vi "FPGA Main V2.vi"() -> ()   [LabVIEW 2018]
doc: "This VI reads all analogue data channels available at the fastest rate supported by the respective hardware and updates a memory address for when each measurement is available.\n\nAt a rate defined by the fastest module (NI 9237 - default of 12.5kHz) this memory is read, combined with the measurements from the 9237 module and written to the FIFO for communication to the RT machine.\n\nThe NI 9237 modeul therefore defines the nominal sampling rate of the system (with slower channels over-sampled).\n\nA time channel (in uSec) is provided with 0 referenced from the first acquisition of the NI 9237 module"
uses:
  <vilib>/LabVIEW Targets/FPGA/cRIO/shared/nicrio_ModuleControls/nicrio_cRIO-9237_DataRatesRing.ctl
  <vilib>/Platform/TimedLoop/XDataNode/timing_clust.ctl
  <vilib>/Platform/TimedLoop/XDataNode/nitl_modes.ctl
  <vilib>/Platform/TimedLoop/XDataNode/wakeup.ctl
  <vilib>/rvi/Emulation/niFpgaGetClockAttributes.vi
  <vilib>/rvi/Emulation/niFpgaSctlEmulationGetInTimedLoop.vi
  <vilib>/rvi/Emulation/niFpgaEmulationReportErrorSimple.vi
  <vilib>/rvi/Emulation/niFpgaProcessEmulError.vi
  <vilib>/rvi/eio/common/nirviEmuTemplatePropertySet_noerrors.vi
  <vilib>/rvi/eio/common/nirviEmuTemplateMethod_errors.vi
  <vilib>/rvi/interface/RandomDataEmulation/niFpgaRandomDataHandleErrors.vi
  <vilib>/rvi/Memory/Memory_Emulation/nirvimemoryFastEmulation.vi
  <vilib>/rvi/Memory/Memory_Emulation/nirvimemoryEmulation.vi
  <vilib>/rvi/Emulation/niFpgaEmulationIsFPGAContextNoSignature.vi
  <vilib>/rvi/DataTransferAndStorage/Container/Common/niFpgaContainerGetUniqueNameForEmu.vi
  <vilib>/rvi/errors/nirviReportUnexpectedCaseInternalError (U32).vi
  <vilib>/rvi/Emulation/niFpgaCriticalErrorInLSC.vi
  <vilib>/eio/EIOPropertyNode/EIOPropertyNode.xnode
  <vilib>/eio/EIONode/EIONode.xnode
  <vilib>/rvi/DataTransferAndStorage/Container/XNode/niFpgaContainer.xnode
  <vilib>/rvi/interface/RandomDataEmulation/nirviRandomDataFpgaReadWriteTemplate.vi
  <vilib>/platform/TimedLoop/XDataNode/XDataNode.xnode
  <vilib>/eio/EIOMethodNode/EIOMethodNode.xnode
  <vilib>/Platform/TimedLoop/XDataNode/XDNodeRunTimeDep.lvlib
  <vilib>/rvi/eio/common/nirviEmuTemplatePropertyGet_errors.vi
  <vilib>/rvi/eio/common/nirviEmuTemplatePropertyGet_noerrors.vi
  <vilib>/rvi/eio/common/nirviEmuTemplatePropertySet_errors.vi
panel:
  in  "speedDirection":bool=TRUE
  in  "speed filter":u16=150
  in  "switch encoders":bool
  in  "falling edge (F)":bool caption="Torque encoder direction"
  in  "filterTorque":bool
  in  "Data Rate":T1=1 items=["50.000 kS/s (NI 9237)"=1, "25.000 kS/s (NI 9237)"=2, "16.667 kS/s (NI 9237)"=3, "12.500 kS/s (NI 9237)"=4, "10.000 kS/s (NI 9237)"=5, "8.333 kS/s (NI 9237)"=6, "7.143 kS/s (NI 9237)"=7, "6.250 kS/s (NI 9237)"=8, "5.556 kS/s (NI 9237)"=9, "5.000 kS/s (NI 9237)"=10, "4.545 kS/s (NI 9237)"=11, "4.167 kS/s (NI 9237)"=12, "3.846 kS/s (NI 9237)"=13, "3.571 kS/s (NI 9237)"=14, "3.333 kS/s (NI 9237)"=15, "3.125 kS/s (NI 9237)"=16, "2.941 kS/s (NI 9237)"=17, "2.778 kS/s (NI 9237)"=18, "2.632 kS/s (NI 9237)"=19, "2.500 kS/s (NI 9237)"=20, "2.381 kS/s (NI 9237)"=21, "2.273 kS/s (NI 9237)"=22, "2.174 kS/s (NI 9237)"=23, "2.083 kS/s (NI 9237)"=24, "2.000 kS/s (NI 9237)"=25, "1.923 kS/s (NI 9237)"=26, "1.852 kS/s (NI 9237)"=27, "1.786 kS/s (NI 9237)"=28, "1.724 kS/s (NI 9237)"=29, "1.667 kS/s (NI 9237)"=30, "1.613 kS/s (NI 9237)"=31]
  in  "encoders offset":sgl caption="encoder offset (radians)"
  out "Total channel count":u32=61
  out "timestamp":u32
  out "FIFO full counter":i32
  in  "Safe Voltage":fxp<+/-,20,5>[](array[numeric])=[0.0, 0.0, 0.0, 0.0]
  in  "Safe Digital":bool[](array[boolean])=[FALSE, FALSE, FALSE, FALSE, FALSE, FALSE, FALSE, FALSE]
  in  "Voltage Out":fxp<+/-,20,5>[](array[numeric])=[0.0, 0.0, 0.0, 0.0]
  in  "Update Outputs":bool
  in  "Mod 8":bool[](array[boolean])=[FALSE, FALSE, FALSE, FALSE, FALSE, FALSE, FALSE, FALSE]
  out "E Stop":bool
  in  "Stop acquire":bool
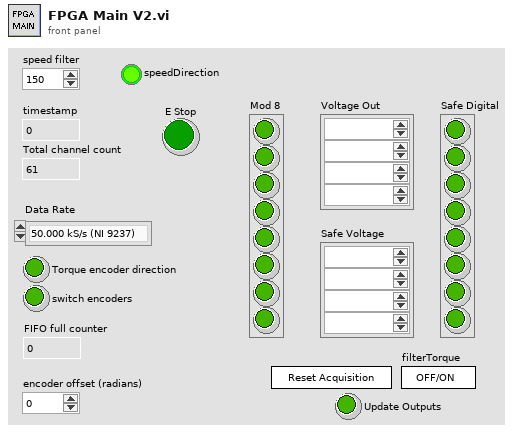
[diagram p1: front panel]
types:
  T1 = typedef "nicrio_cRIO-9237_DataRatesRing.ctl" = u8
  T2 = typedef "XDNodeRunTimeDep.lvlib/timing_clust.ctl" = cluster{"Expected End [f-1]":u64, "Actual End [f-1]":u64, "Finished Late? [f-1]":bool, "Expected End [i-1]":u64, "Actual End [i-1]":u64, "Finished Late? [i-1]":bool, "Expected Start [i]":u64, "Actual Start [i]":u64, "Expected Start [f]":u64, "Actual Start [f]":u64, "Source Name":string, "Structure Name":string, "Period":i64, "Deadline":i64, "Offset":i64, "Start":i64, "Priority":i32, "Timeout":i32, "Mode":T3, "Wakeup Reason":T4, "Error":errorcluster, "Source Type":string, "Secondary Source Type":string, "Global End Time":u64, "Global Start Time":u64, "Frame Duration":u64, "Iteration Duration":u64, "Assigned CPU":i32, "I/O Scan Engine Mode":u32}
  T3 = typedef "XDNodeRunTimeDep.lvlib/nitl_modes.ctl" = enum32{"No Change", "Process missed periods, maintain original phase", "Discard missed periods, maintain original phase", "Process missed periods, ignore original phase", "Discard missed periods, ignore original phase"}
  T4 = typedef "XDNodeRunTimeDep.lvlib/wakeup.ctl" = enum32{"Normal", "Aborted", "Asynchronous wakeup", "Timing source error", "Timed loop error", "Timeout"}
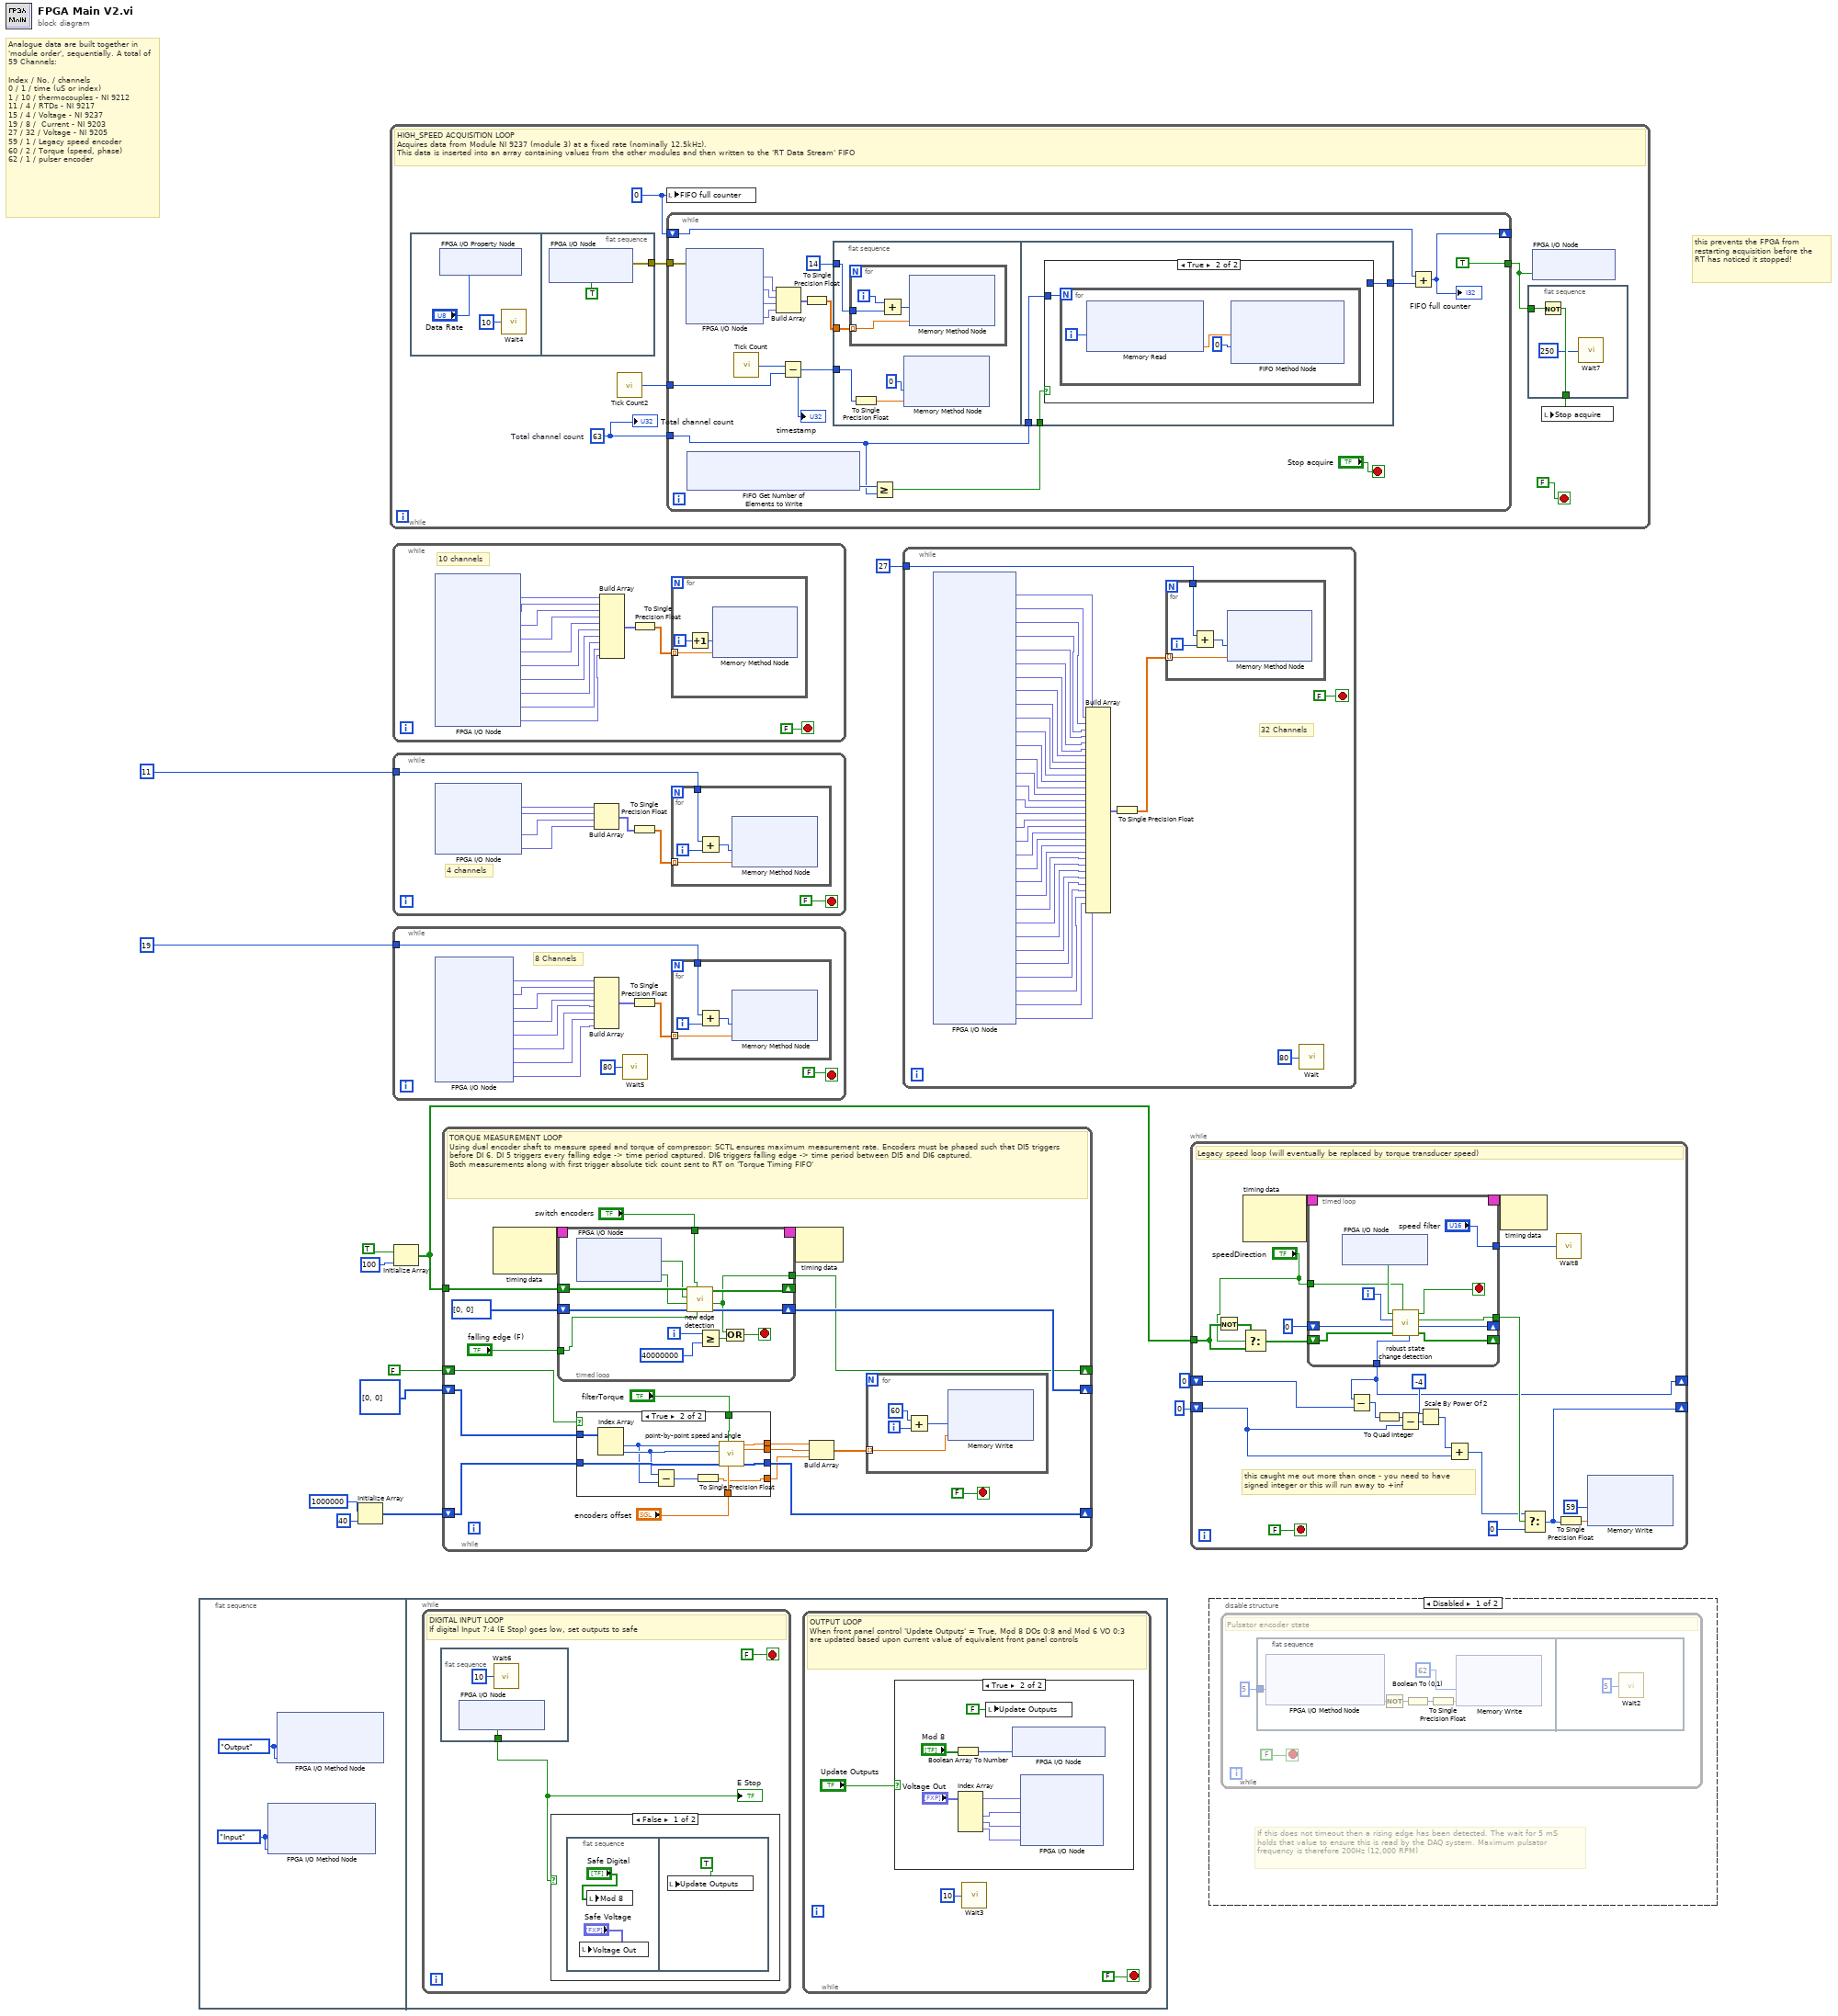
[diagram p0: block diagram]
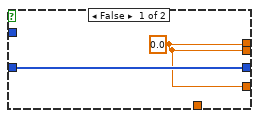
[diagram p5: hidden frame]
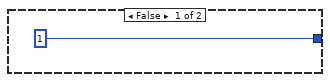
[diagram p6: hidden frame]
diagram:
  # "this prevents the FPGA from restarting acquisition before the RT has noticed it stopped!"
  # "Analogue data are built together in 'module order', sequentially. A total of 59 Channels:\n\nIndex / No. / channels\n0 / 1 / time (uS or index)\n1 / 10 / thermocouples - NI 9212\n11 / 4 / RTDs - NI 9217\n15 / 4 / Voltage - NI 9237\n19 / 8 /  Current - NI 9203\n27 / 32 / Voltage - NI 9205\n59 / 1 / Legacy speed encoder\n60 / 2 / Torque (speed, phase)\n62 / 1 / pulser encoder"
  n1 = flat-sequence {
    frame #0 {
      w14 = enum8{"No Change", "Input", "Output"}."Output" ("DIO 7:4")
      w15 = enum8{"No Change", "Input", "Output"}."Input" ("DIO 7:4")
      n2 = xnode "FPGA I/O Method Node"("DIO 7:4"=w15, "DIO 3:0"=w15) -> ()  [unwired: 1 in, 1 out]
      n3 = xnode "FPGA I/O Method Node"("DIO 7:4"=w14, "DIO 3:0"=w14) -> ()  [unwired: 1 in, 1 out]
    }
    frame #1 {
      n4 = while {
        stop <- FALSE stop-if-true
        # "DIGITAL INPUT LOOP\nIf digital Input 7:4 (E Stop) goes low, set outputs to safe"
        n5 = flat-sequence {
          tunnel: [w30] -> w27
          frame #0 {
            n6 = xnode "FPGA I/O Node"() -> ("Mod7/DIO4"=w30:bool)  [unwired: 1 in, 1 out]
            n7 = call "Wait6"("Count(uSec)"=u8 10) -> ()  [unwired: 1 out]
          }
        }
        n8 = case shown="False" w27 {
          frame False {
            n9 = flat-sequence {
              frame #0 {
                n10 = local write "Voltage Out"("Safe Voltage") -> ()
                n11 = local write "Mod 8"("Safe Digital") -> ()
              }
              frame #1 {
                n12 = local write "Update Outputs"(TRUE ("Update Outputs")) -> ()
              }
            }
          }
          frame True {
          }
        }
        "E Stop" <- w27
      }
      n13 = while {
        stop <- FALSE stop-if-true
        # "OUTPUT LOOP\nWhen front panel control 'Update Outputs' = True, Mod 8 DOs 0:8 and Mod 6 VO 0:3 are updated based upon current value of equivalent front panel controls"
        n14 = case shown="True" "Update Outputs" {
          frame False {
          }
          frame True {
            n15 = Boolean Array To Number(Boolean array="Mod 8") -> (number=w25:u8)
            n16 = Index Array(array="Voltage Out") -> (element #1=w23:fxp<+/-,20,5>, element #2=w22:fxp<+/-,20,5>, element #3=w21:fxp<+/-,20,5>, element #4=w20:fxp<+/-,20,5>)  [unwired: 4 in]
            n17 = local write "Update Outputs"(FALSE ("Update Outputs")) -> ()
            n18 = xnode "FPGA I/O Node"("Mod8/DIO7:0"=w25) -> ()  [unwired: 1 in, 1 out]
            n19 = xnode "FPGA I/O Node"("Mod6/AO0"=w23, "Mod6/AO1"=w22, "Mod6/AO2"=w21, "Mod6/AO3"=w20) -> ()  [unwired: 4 in, 4 out]
          }
        }
        n20 = call "Wait3"("Count(uSec)"=u16 10 ("Count(Ticks)")) -> ()  [unwired: 1 out]
      }
    }
  }
  n21 = Initialize Array(u32 1000000 ("64bit integer"), 40 ("dimension size")) -> (w8:u32[])
  n22 = while {
    stop <- FALSE stop-if-true
    w35 = 0 ("FIFO full counter")
    w38 = u32 63  # Total channel count
    # "HIGH_SPEED ACQUISITION LOOP\nAcquires data from Module NI 9237 (module 3) at a fixed rate (nominally 12.5kHz).\nThis data is inserted into an array containing values from the other modules and then written to the 'RT Data Stream' FIFO"
    n23 = flat-sequence {
      tunnel: [w47] -> w39
      frame #0 {
        n24 = xnode "FPGA I/O Property Node"("Data Rate"="Data Rate") -> ()  [unwired: 1 in, 1 out]
        n25 = call "Wait4"("Count(mSec)"=u16 10) -> ()  [unwired: 1 out]
      }
      frame #1 {
        n26 = xnode "FPGA I/O Node"("Mod3/Start"=TRUE) -> ("error out"=w47:errorcluster)  [unwired: 2 in, 1 out]
      }
    }
    n27 = call "Tick Count2"() -> ("Tick Count(uSec)"=w40:u32)
    n28 = local write "FIFO full counter"(w35) -> ()
    n29 = while {
      tunnel: [TRUE ("I/O Item")] -> w37
      tunnel: w39 -> [w65]
      tunnel: w38 -> [w50]
      shift-right: [w58] -> _
      shift-left: w35 -> [w56]
      tunnel: w40 -> [w59]
      stop <- "Stop acquire" stop-if-true
      n30 = xnode "FPGA I/O Node"("error in"=w65) -> ("Mod3/AI0"=w64:fxp<+/-,24,-4>, "Mod3/AI1"=w63:fxp<+/-,24,-4>, "Mod3/AI2"=w62:fxp<+/-,24,-4>, "Mod3/AI3"=w61:fxp<+/-,24,-4>)  [unwired: 4 in, 5 out]
      n31 = xnode ("FIFO Get Number of Elements to Write")() -> ("Number of Elements to Write"=w52:u32)  [unwired: 1 in, 1 out]
      n32 = call "Tick Count"() -> ("Tick Count(uSec)"=w55:u32)
      n33 = Build Array(w64, w63, w62, w61) -> (w60:fxp<+/-,24,-4>[])
      n34 = Subtract(x=w55, y=w59) -> (x-y=w48:u32)
      "timestamp" <- w48
      n35 = To Single Precision Float(number=w60) -> (single precision float=w54:sgl[])
      n36 = flat-sequence {
        tunnel: w54 -> [w71]
        tunnel: 14 ("index") -> [w70]
        tunnel: w48 -> [w68]
        tunnel: w50 -> [w78]
        tunnel: [w77] -> w49
        tunnel: w51 -> [w76]
        frame #0 {
          n37 = for {
            tunnel: w71 -> [w75] mode=indexing
            tunnel: w70 -> [w74]
            i -> [w72]
            n38 = Add(x=w72, y=w74) -> (x+y=w73:i32)
            n39 = xnode ("Memory Method Node")("Address"=w73, "Data"=w75) -> ()  [unwired: 1 in, 1 out]
          }
          n40 = To Single Precision Float(number=w68) -> (single precision float=w69:sgl)
          n41 = xnode ("Memory Method Node")("Address"=u32 0, "Data"=w69) -> ()  [unwired: 1 in, 1 out]
        }
        frame #1 {
          n42 = case shown="True" w76 {
            tunnel: [1 _] -> w77
            tunnel: w78 -> [_ w80]
            frame False {
            }
            frame True {
              n43 = for {
                N: w80 -> [_]
                i -> [w81]
                n44 = xnode ("Memory Read")("Address"=w81) -> ("Data"=w82:sgl)  [unwired: 1 in, 1 out]
                n45 = xnode ("FIFO Method Node")("Element"=w82, "Timeout"=0) -> ()  [unwired: 1 in, 2 out]
              }
            }
          }
        }
      }
      n46 = Greater Or Equal?(x=w52, y=w50) -> (x >= y?=w51:bool)
      n47 = Add(x=w56, y=w49) -> (x+y=w58:i32)
      "FIFO full counter" <- w58
    }
    n48 = flat-sequence {
      tunnel: w37 -> [w43]
      tunnel: [w42] -> w34
      frame #0 {
        n49 = Not(x=w43) -> (.not. x?=w42:bool)
        n50 = call "Wait7"("Count(mSec)"=u8 250) -> ()  [unwired: 1 out]
      }
    }
    n51 = xnode "FPGA I/O Node"("Mod3/Stop"=w37) -> ()  [unwired: 1 in, 1 out]
    n52 = local write "Stop acquire"(w34) -> ()
    "Total channel count" <- w38
  }
  n53 = while {
    stop <- FALSE stop-if-true
    # "10 channels"
    n54 = xnode "FPGA I/O Node"() -> ("Mod1/TC0"=w96:fxp<+/-,24,-2>, "Mod1/TC1"=w95:fxp<+/-,24,-2>, "Mod1/TC2"=w94:fxp<+/-,24,-2>, "Mod1/TC3"=w93:fxp<+/-,24,-2>, "Mod1/TC4"=w92:fxp<+/-,24,-2>, "Mod1/TC5"=w91:fxp<+/-,24,-2>, "Mod1/TC6"=w90:fxp<+/-,24,-2>, "Mod1/TC7"=w89:fxp<+/-,24,-2>, "Mod1/CJC0"=w86:fxp<+/-,24,-2>, "Mod1/CJC1"=w85:fxp<+/-,24,-2>)  [unwired: 10 in, 10 out]
    n55 = Build Array(w96, w95, w94, w93, w92, w91, w90, w89, w86, w85) -> (w88:fxp<+/-,24,-2>[])
    n56 = To Single Precision Float(number=w88) -> (single precision float=w87:sgl[])
    n57 = for {
      tunnel: w87 -> [w99] mode=indexing
      i -> [w98]
      n58 = Increment(x=w98) -> (x+1=w97:i32)
      n59 = xnode ("Memory Method Node")("Address"=w97, "Data"=w99) -> ()  [unwired: 1 in, 1 out]
    }
  }
  n60 = while {
    tunnel: 11 ("Numeric") -> [w101]
    stop <- FALSE stop-if-true
    # "4 channels"
    n61 = xnode "FPGA I/O Node"() -> ("Mod2/RTD0"=w107:fxp<+/-,24,10>, "Mod2/RTD1"=w106:fxp<+/-,24,10>, "Mod2/RTD2"=w105:fxp<+/-,24,10>, "Mod2/RTD3"=w102:fxp<+/-,24,10>)  [unwired: 4 in, 4 out]
    n62 = Build Array(w107, w106, w105, w102) -> (w104:fxp<+/-,24,10>[])
    n63 = To Single Precision Float(number=w104) -> (single precision float=w103:sgl[])
    n64 = for {
      tunnel: w103 -> [w111] mode=indexing
      tunnel: w101 -> [w108]
      i -> [w110]
      n65 = Add(x=w108, y=w110) -> (x+y=w109:i32)
      n66 = xnode ("Memory Method Node")("Address"=w109, "Data"=w111) -> ()  [unwired: 1 in, 1 out]
    }
  }
  n67 = while {
    tunnel: 19 ("Numeric") -> [w118]
    stop <- FALSE stop-if-true
    # "8 Channels"
    n68 = xnode "FPGA I/O Node"() -> ("Mod4/AI0"=w124:fxp<+/-,21,-4>, "Mod4/AI1"=w123:fxp<+/-,21,-4>, "Mod4/AI2"=w122:fxp<+/-,21,-4>, "Mod4/AI3"=w119:fxp<+/-,21,-4>, "Mod4/AI4"=w117:fxp<+/-,21,-4>, "Mod4/AI5"=w116:fxp<+/-,21,-4>, "Mod4/AI6"=w115:fxp<+/-,21,-4>, "Mod4/AI7"=w114:fxp<+/-,21,-4>)  [unwired: 8 in, 8 out]
    n69 = Build Array(w124, w123, w122, w119, w117, w116, w115, w114) -> (w121:fxp<+/-,21,-4>[])
    n70 = call "Wait5"("Count(uSec)"=u8 80) -> ()  [unwired: 1 out]
    n71 = To Single Precision Float(number=w121) -> (single precision float=w120:sgl[])
    n72 = for {
      tunnel: w120 -> [w128] mode=indexing
      tunnel: w118 -> [w125]
      i -> [w127]
      n73 = Add(x=w125, y=w127) -> (x+y=w126:i32)
      n74 = xnode ("Memory Method Node")("Address"=w126, "Data"=w128) -> ()  [unwired: 1 in, 1 out]
    }
  }
  n75 = Initialize Array(TRUE, 100 ("edge buffer size")) -> (w4:bool[])
  n76 = while {
    shift-right: [w145] -> _
    shift-left: w8 -> [w146]
    tunnel: w4 -> [w144]
    shift-right: [w132] -> _
    shift-left: u32[] [0, 0] ("step") -> [w131]
    shift-right: [w129] -> _
    shift-left: FALSE ("edge detected") -> [w130]
    stop <- FALSE stop-if-true
    # "TORQUE MEASUREMENT LOOP\nUsing dual encoder shaft to measure speed and torque of compressor: SCTL ensures maximum measurement rate. Encoders must be phased such that DI5 triggers before DI 6. DI 5 triggers every falling edge -> time period captured. DI6 triggers falling edge -> time period between DI5 and DI6 captured.\nBoth measurements along with first trigger absolute tick count sent to RT on 'Torque Timing FIFO'"
    n77 = node-c288() -> (w142:T2)  [unwired: 2 in]
    n78 = timed-loop {
      timing: w142 -> [_]
      timing-out: [_] -> w141
      shift-right: [w171] -> _
      shift-left: w144 -> [w174]
      shift-right: [w172] -> w132
      shift-left: u32[] [0, 0] ("step") -> [w173]
      tunnel: "falling edge (F)" -> [w168]
      tunnel: [w169] -> w129
      tunnel: "switch encoders" -> [w165]
      i -> [w177]
      stop <- w170 stop-if-true
      n79 = xnode "FPGA I/O Node"() -> ("Mod7/DIO0"=w167:bool, "Mod7/DIO1"=w166:bool)  [unwired: 2 in, 2 out]
      n80 = call "new edge detection.vi"("rising edge (T)"=w168, "switch encoders (F)"=w165, "ticks"=w173, "encoder 2"=w166, "encoder 1"=w167, "history in"=w174) -> ("ticks out"=w172:u32[], "edge detected"=w169:bool, "history out"=w171:bool[])  [unwired: 3 in]
      n81 = Greater Or Equal?(x=w177, y=40000000) -> (x >= y?=w175:bool)
      n82 = Or(x=w169, y=w175) -> (x .or. y?=w170:bool)
    }
    n83 = case shown="True" w130 {
      tunnel: w146 -> [w149 w160]
      tunnel: [w149 w159] -> w145
      tunnel: [w148 w158] -> w138
      tunnel: [w148 w157] -> w134
      tunnel: w131 -> [_ w156]
      tunnel: "encoders offset" -> [_ w155]
      tunnel: "filterTorque" -> [_ w154]
      tunnel: [w148 w150] -> w133
      frame False {
        w148 = sgl 0.0 ("calculated speed (Hz)")
      }
      frame True {
        n84 = Index Array(array=w156) -> (element #1=w152:u32, element #2=w153:u32)  [unwired: 2 in]
        n85 = Subtract(x=w153, y=w152) -> (x-y=w151:u32)
        n86 = To Single Precision Float(number=w151) -> (single precision float=w150:sgl)
        n87 = call "point-by-point speed and angle.vi"("encoder fixed offest"=w155, "filter torque"=w154, "speed history in"=w160, "angle pulse"=w153, "speed pulse"=w152) -> ("speed history out"=w159:u32[], "calculated angle (radians)"=w157:sgl, "calculated speed (rad/tick)"=w158:sgl)  [unwired: 4 in]
      }
    }
    n88 = node-c288(w141) -> ()  [unwired: 1 out]
    n89 = Build Array(w138, w134, w133) -> (w137:sgl[])
    n90 = for {
      tunnel: w137 -> [w161] mode=indexing
      i -> [w162]
      n91 = Add(x=u32 60 ("Address"), y=w162) -> (x+y=w163:u32)
      n92 = xnode ("Memory Write")("Address"=w163, "Data"=w161) -> ()  [unwired: 1 in, 1 out]
    }
  }
  n93 = while {
    tunnel: 27 ("Numeric") -> [w217]
    stop <- FALSE stop-if-true
    # "32 Channels"
    n94 = xnode "FPGA I/O Node"() -> ("Mod5/AI0"=w185:fxp<+/-,26,5>, "Mod5/AI1"=w186:fxp<+/-,26,5>, "Mod5/AI2"=w187:fxp<+/-,26,5>, "Mod5/AI3"=w188:fxp<+/-,26,5>, "Mod5/AI4"=w189:fxp<+/-,26,5>, "Mod5/AI5"=w190:fxp<+/-,26,5>, "Mod5/AI6"=w191:fxp<+/-,26,5>, "Mod5/AI7"=w192:fxp<+/-,26,5>, "Mod5/AI8"=w216:fxp<+/-,26,5>, "Mod5/AI9"=w215:fxp<+/-,26,5>, "Mod5/AI10"=w214:fxp<+/-,26,5>, "Mod5/AI11"=w213:fxp<+/-,26,5>, "Mod5/AI12"=w212:fxp<+/-,26,5>, "Mod5/AI13"=w211:fxp<+/-,26,5>, "Mod5/AI14"=w210:fxp<+/-,26,5>, "Mod5/AI15"=w209:fxp<+/-,26,5>, "Mod5/AI16"=w208:fxp<+/-,26,5>, "Mod5/AI17"=w207:fxp<+/-,26,5>, "Mod5/AI18"=w206:fxp<+/-,26,5>, "Mod5/AI19"=w205:fxp<+/-,26,5>, "Mod5/AI20"=w204:fxp<+/-,26,5>, "Mod5/AI21"=w203:fxp<+/-,26,5>, "Mod5/AI22"=w202:fxp<+/-,26,5>, "Mod5/AI23"=w201:fxp<+/-,26,5>, "Mod5/AI24"=w200:fxp<+/-,26,5>, "Mod5/AI25"=w199:fxp<+/-,26,5>, "Mod5/AI26"=w198:fxp<+/-,26,5>, "Mod5/AI27"=w197:fxp<+/-,26,5>, "Mod5/AI28"=w196:fxp<+/-,26,5>, "Mod5/AI29"=w195:fxp<+/-,26,5>, "Mod5/AI30"=w194:fxp<+/-,26,5>, "Mod5/AI31"=w193:fxp<+/-,26,5>)  [unwired: 32 in, 32 out]
    n95 = Build Array(w185, w186, w187, w188, w189, w190, w191, w192, w216, w215, w214, w213, w212, w211, w210, w209, w208, w207, w206, w205, w204, w203, w202, w201, w200, w199, w198, w197, w196, w195, w194, w193) -> (w218:fxp<+/-,26,5>[])
    n96 = To Single Precision Float(number=w218) -> (single precision float=w184:sgl[])
    n97 = for {
      tunnel: w184 -> [w222] mode=indexing
      tunnel: w217 -> [w219]
      i -> [w221]
      n98 = Add(x=w219, y=w221) -> (x+y=w220:i32)
      n99 = xnode ("Memory Method Node")("Address"=w220, "Data"=w222) -> ()  [unwired: 1 in, 1 out]
    }
    n100 = call "Wait"("Count(uSec)"=u8 80) -> ()  [unwired: 1 out]
  }
  n101 = while {
    shift-right: [w233] -> _
    shift-left: i64 0 -> [w239]
    tunnel: w4 -> [w225]
    shift-right: [w229] -> _
    shift-left: u32 0 ("tick") -> [w228]
    stop <- FALSE stop-if-true
    # "this caught me out more than once - you need to have signed integer or this will run away to +inf"
    # "Legacy speed loop (will eventually be replaced by torque transducer speed)"
    n102 = Not(x=w225) -> (.not. x?=w226:bool[])
    n103 = node-c288() -> (w245:T2)  [unwired: 2 in]
    n104 = Select(t=w226, s="speedDirection", f=w225) -> (s? t:f=w224:bool[])
    n105 = timed-loop {
      timing: w245 -> [_]
      timing-out: [_] -> w244
      shift-right: [w253] -> _
      shift-left: i16 0 ("step") -> [w254]
      tunnel: [w251] -> w234
      tunnel: [w250] -> w229
      shift-right: [w248] -> _
      shift-left: w224 -> [w249]
      tunnel: ["speed filter"] -> w227
      tunnel: "speedDirection" -> [w246]
      i -> [w255]
      stop <- w252 stop-if-true
      n106 = xnode "FPGA I/O Node"() -> ("Mod7/DIO3"=w256:bool)  [unwired: 1 in, 1 out]
      n107 = call "robust state change detection.vi"("falling edge (F)"=w246, "history"=w249, "step"=w254, "tick"=w255, "New state"=w256) -> ("history out"=w248:bool[], "step out"=w253:i16, "edge detected"=w251:bool, "Stop?"=w252:bool, "tick"=w250:u32)  [unwired: 2 in]
    }
    n108 = Subtract(x=w229, y=w228) -> (x-y=w230:u32)
    n109 = To Quad Integer(1:w230) -> (0:w236:i64)
    n110 = Subtract(x=w236, y=w239) -> (x-y=w240:i64)
    n111 = Scale By Power Of 2(n=i16 -4, x=w240) -> (x*2^n=w242:i64)
    n112 = Add(x=w242, y=w239) -> (x+y=w231:i64)
    n113 = node-c288(w244) -> ()  [unwired: 1 out]
    n114 = Select(t=w231, s=w234, f=u32 0 ("t")) -> (s? t:f=w233:i64)
    n115 = call "Wait8"("Count(uSec)"=w227) -> ()  [unwired: 1 out]
    n116 = To Single Precision Float(number=w233) -> (single precision float=w238:sgl)
    n117 = xnode ("Memory Write")("Address"=u32 59, "Data"=w238) -> ()  [unwired: 1 in, 1 out]
  }
  n118 = disable-structure shown="Disabled" {
    frame Disabled {
      # "If this does not timeout then a rising edge has been detected. The wait for 5 mS holds that value to ensure this is read by the DAQ system. Maximum pulsator frequency is therefore 200Hz (12,000 RPM)"
      n119 = while {
        stop <- FALSE stop-if-true
        # "Pulsator encoder state"
        n120 = flat-sequence {
          tunnel: 5 ("Timeout") -> [w265]
          frame #0 {
            n121 = xnode "FPGA I/O Method Node"("Timeout"=w265) -> ("Timed Out"=w264:bool)  [unwired: 1 in, 1 out]
            n122 = Not(x=w264) -> (.not. x?=w263:bool)
            n123 = Boolean To (0,1)(Boolean=w263) -> (0, 1=w268:i16)
            n124 = To Single Precision Float(number=w268) -> (single precision float=w267:sgl)
            n125 = xnode ("Memory Write")("Address"=u32 62, "Data"=w267) -> ()  [unwired: 1 in, 1 out]
          }
          frame #1 {
            n126 = call "Wait2"("Count(mSec)"=u16 5 ("Count(uSec)")) -> ()  [unwired: 1 out]
          }
        }
      }
    }
    frame Enabled {
    }
  }
